vi "Stop Vision.vi"(8 "error in (no error)":errorcluster, 11 "Vision Receiver in":refnum<class "Vision Receiver.lvclass">) -> (0 "error out":errorcluster, 3 "Vision Receiver out":refnum<class "Vision Receiver.lvclass">)   [LabVIEW 2022 SP3]
uses:
  Vision Receiver.lvclass
  Vision Receiver.lvclass/Vision Receiver.ctl
  <vilib>/ActorFramework/Message Enqueuer/Message Enqueuer.lvclass/Message Enqueuer.ctl
  <vilib>/ActorFramework/Message Enqueuer/Enqueue.vi
  UDP Reader/UDP Reader Messages/Halt Msg/Halt Msg.lvclass
  C:/Program Files (x86)/National Instruments/LabVIEW 2022/vi.lib/ActorFramework/Message/Message.lvclass
  <vilib>/ActorFramework/Message Priority Queue/Priority Enqueue.vi
  C:/Program Files (x86)/National Instruments/LabVIEW 2022/vi.lib/MGI/Monitored Actor/Monitored Actor/Monitored Actor/Monitored Actor.lvclass
  C:/Program Files (x86)/National Instruments/LabVIEW 2022/vi.lib/ActorFramework/Actor/Actor.lvclass
  C:/Users/ebert/Documents/codes/ssl/repo/Phoenix Reborn/Vision Receiver/Vision Receiver/Vision Receiver.lvclass
  C:/Users/ebert/Documents/codes/ssl/repo/Phoenix Reborn/UDP Data Receiver/UDP Data Receiver/UDP Data Receiver.lvclass
  <vilib>/ActorFramework/Message Enqueuer/Message Enqueuer.lvclass
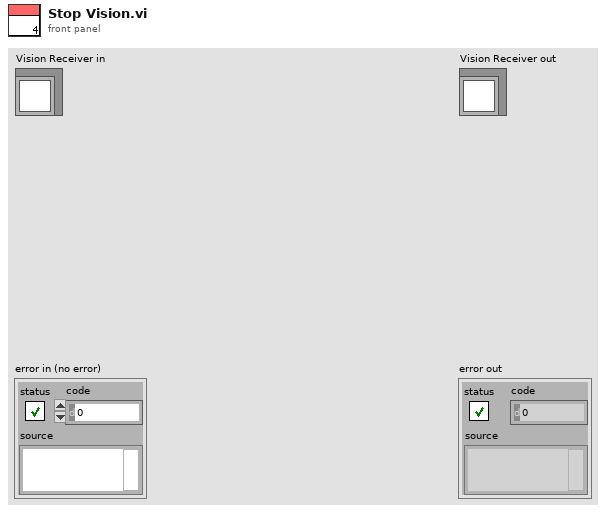
[diagram p1: front panel]
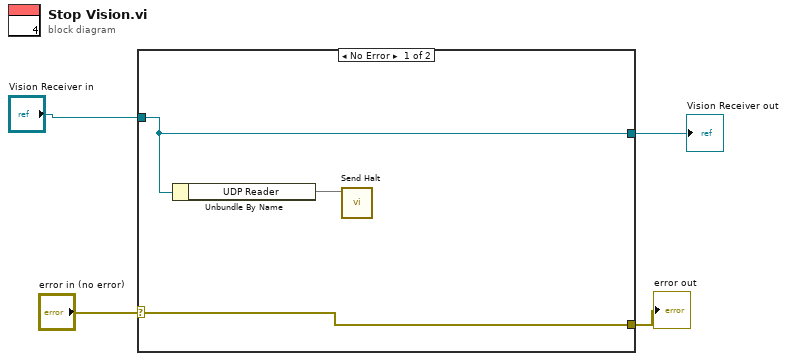
[diagram p0: block diagram]
diagram:
  n1 = case shown="No Error" "error in (no error)" {
    selector: "error in (no error)" -> [w5 w9]
    tunnel: [w5 w9] -> w3
    tunnel: "Vision Receiver in" -> [w7 w8]
    tunnel: [w7 w8] -> w1
    frame No Error {
      n2 = Unbundle By Name(w7) -> ("UDP Reader"=w6)
      n3 = call "Send Halt.vi"("Message Enqueuer"=w6) -> ()  [unwired: 9 in, 2 out]
    }
    frame Error {
    }
  }
  "error out" <- w3
  "Vision Receiver out" <- w1
